vi "Humidity (SubVI).vi"(11 "Waveform":dbl) -> (3 "Numeric":dbl)   [LabVIEW 2022 SP3]
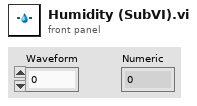
[diagram p1: front panel]
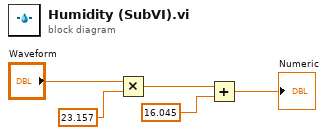
[diagram p0: block diagram]
diagram:
  n1 = Multiply(x="Waveform", y=23.157) -> (x*y=w3:dbl)
  n2 = Add(x=w3, y=16.045) -> (x+y=→"Numeric":dbl)
